vi "configure tdms file properties.vi"(8 "error in (no error)":errorcluster, 9 "property values":variant[](array[variant]), 10 "property names":string[](array[string]), 11 "tdms file":refnum<k34>) -> (0 "error out":errorcluster, 3 "tdms file out":refnum<k34>)   [LabVIEW 2015, in "TDMS datalogger runtime.lvclass"]
uses:
  TDMS datalogger runtime.lvclass
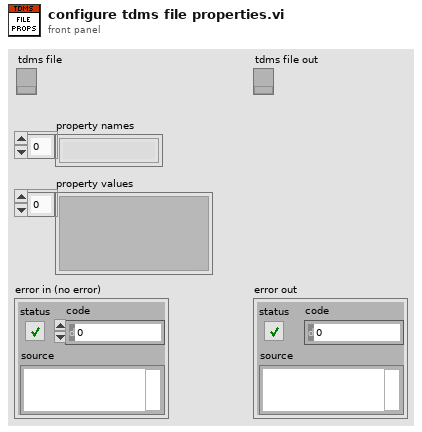
[diagram p1: front panel]
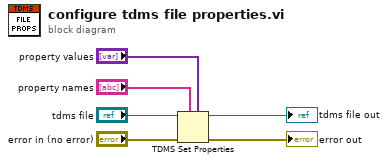
[diagram p0: block diagram]
diagram:
  n1 = TDMS Set Properties(5:"property values", 7:"property names", 8:"error in (no error)", 11:"tdms file") -> (0:→"error out":errorcluster, 3:→"tdms file out":refnum<k34>)  [unwired: 2 in, 2 out]
